vi "Wait_Return_IHM.vi"(8 "error in (no error)":errorcluster caption="entrée d'erreur (pas d'erreur)", 11 "Class Popup (Default) en entrée":refnum<class "Popup Autotest_Without_Actor.lvclass">) -> (0 "error out":errorcluster caption="sortie d'erreur", 3 "Class Popup (Default) en sortie":refnum<class "Popup Autotest_Without_Actor.lvclass">)   [LabVIEW 2020, in "Library Instrument & Equipement.lvlib" / "Library Popup.lvlib" / "Popup Autotest_Without_Actor.lvclass"]
uses:
  Popup Autotest_Without_Actor.lvclass
  C:/Users/ngarcin/OneDrive - Altyor/Standard TB/Class/Popup/Class Popup Autotest (Default)/Popup Autotest (Default).lvclass
  Variable Instr.vi
  Class Popup Autotest (Default)/Popup Autotest (Default).lvclass
  Popup Autotest_Without_Actor.lvclass/Popup Autotest_Without_Actor.ctl
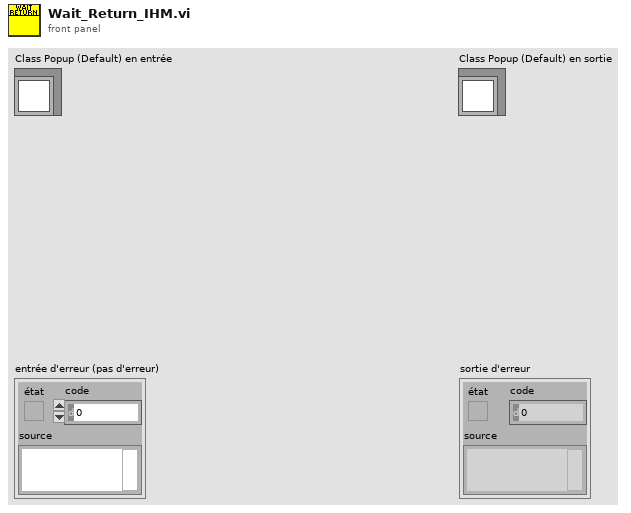
[diagram p1: front panel]
types:
  T1 = cluster{"Name":string, "Instrument":refnum<class "Class Instrument (Default).lvclass">, "Close After Autotest":bool}[]
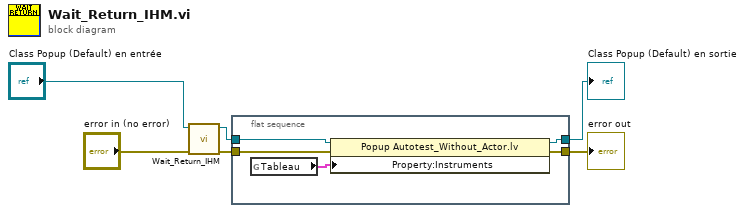
[diagram p0: block diagram]
diagram:
  n1 = call-parent "Wait_Return_IHM.vi"("error in (no error)"="error in (no error)", "Class Popup (Default) en entrée"="Class Popup (Default) en entrée") -> ("error out"=w1:errorcluster, "Class Popup (Default) en sortie"=w4:refnum<class "Popup Autotest_Without_Actor.lvclass">)  [unwired: 8 in]
  n2 = flat-sequence {
    tunnel: w4 -> [w11]
    tunnel: [w10] -> w3
    tunnel: [w9] -> w2
    tunnel: w1 -> [w8]
    frame #0 {
      n3 = global read "Variable Instr.vi" "Tableau"() -> (w7:T1)
      n4 = property class="Popup Autotest_Without_Actor.lv"(reference=w11, error in=w8, "Property:Instruments"=w7) -> (reference out=w10:refnum<class "Popup Autotest_Without_Actor.lvclass">, error out=w9:errorcluster)
    }
  }
  "error out" <- w2
  "Class Popup (Default) en sortie" <- w3
